vi "REST_req.vi"(5 "Request":T2(ring), 6 "Multipart Data In":T1[](array[typedef])=[{"Name"="imageblock1", "Value"="Collectable", "File"=path "C:/Users/monke/Desktop/Work/VIs to modify/ONENOTE/Sandbox/curl-logo.png", "Filename"="curl-logo.png", "MIME type"="image/png"}, {"Name"="content", "Value"="swagmaster flash", "File"=path "", "Filename"="Nothing", "MIME type"="image/png"}], 7 "Headers":string, 8 "error in":errorcluster, 9 "Body":string, 10 "Content-Type":string, 11 "URL":string) -> (0 "error out":errorcluster, 2 "ERROR":string, 3 "OUTPUT":string)   [LabVIEW 2016]
uses:
  <vilib>/httpClient/MultipartData.ctl
  <vilib>/httpClient/LabVIEWHTTPClient.lvlib
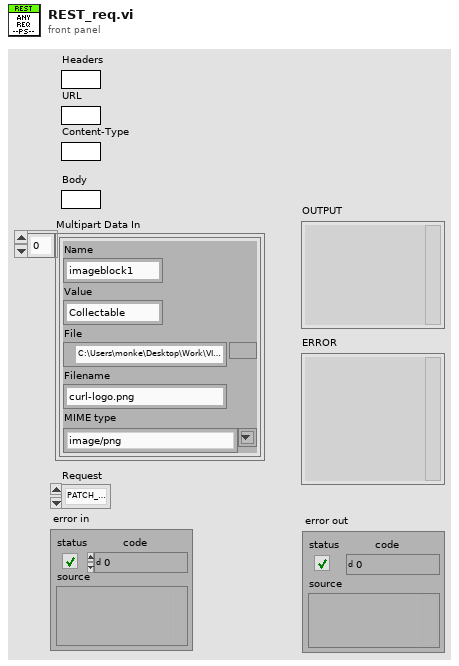
[diagram p1: front panel]
types:
  T1 = typedef "LabVIEWHTTPClient.lvlib/MultipartData.ctl" = cluster{"Name":string, "Value":string, "File":path, "Filename":string, "MIME type":string}
  T2 = enum16{"PATCH_MULTIPART", "POST_MULTIPART", "PATCH", "DELETE", "HEAD", "PUT", "GET"}
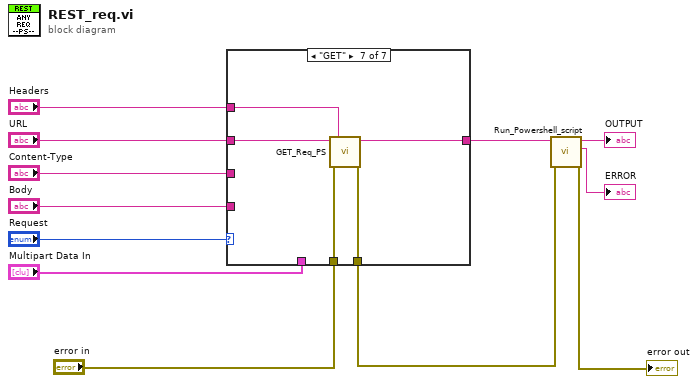
[diagram p0: block diagram]
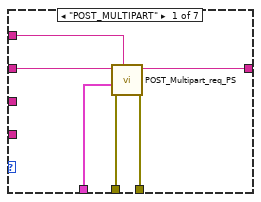
[diagram p2: hidden frame]
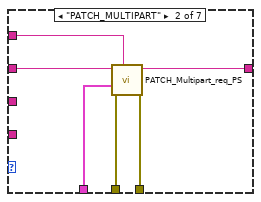
[diagram p3: hidden frame]
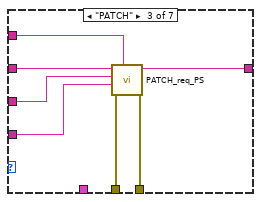
[diagram p4: hidden frame]
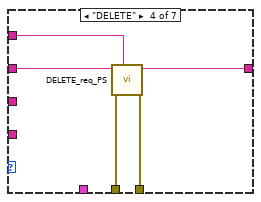
[diagram p5: hidden frame]
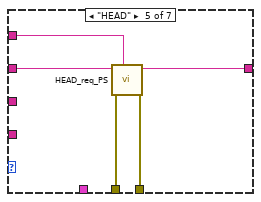
[diagram p6: hidden frame]
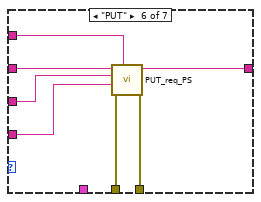
[diagram p7: hidden frame]
diagram:
  n1 = case shown="\"GET\"" "Request" {
    tunnel: "Multipart Data In" -> [w18 w24 _ _ _ _ _]
    tunnel: "URL" -> [w15 w23 w31 w33 w39 w48 w50]
    tunnel: "error in" -> [w17 w19 w30 w36 w41 w45 w51]
    tunnel: [w16 w20 w29 w35 w40 w44 w52] -> w5
    tunnel: "Headers" -> [w14 w22 w28 w32 w38 w43 w49]
    tunnel: [w13 w21 w25 w34 w37 w42 w53] -> w6
    tunnel: "Content-Type" -> [_ _ w26 _ _ w47 _]
    tunnel: "Body" -> [_ _ w27 _ _ w46 _]
    frame "POST_MULTIPART" {
      n2 = call "POST_Multipart_req_PS.vi"("Headers"=w14, "error in"=w17, "Multipart Data In"=w18, "URL"=w15) -> ("error out"=w16:errorcluster, "Multipart PATCH Request"=w13:string)  [unwired: 6 in]
    }
    frame "PATCH_MULTIPART" {
      n3 = call "PATCH_Multipart_req_PS.vi"("Headers"=w22, "error in"=w19, "Multipart Data In"=w24, "URL"=w23) -> ("error out"=w20:errorcluster, "Multipart PATCH Request"=w21:string)  [unwired: 6 in]
    }
    frame "PATCH" {
      n4 = call "PATCH_req_PS.vi"("Headers"=w28, "error in"=w30, "Body"=w27, "ContentType"=w26, "URL"=w31) -> ("error out"=w29:errorcluster, "PATCH Request"=w25:string)  [unwired: 5 in]
    }
    frame "DELETE" {
      n5 = call "DELETE_req_PS.vi"("Headers"=w32, "error in"=w36, "URL"=w33) -> ("error out"=w35:errorcluster, "DELETE Request"=w34:string)  [unwired: 7 in]
    }
    frame "HEAD" {
      n6 = call "HEAD_req_PS.vi"("Headers"=w38, "error in"=w41, "URL"=w39) -> ("error out"=w40:errorcluster, "HEAD Request"=w37:string)  [unwired: 7 in]
    }
    frame "PUT" {
      n7 = call "PUT_req_PS.vi"("Headers"=w43, "error in"=w45, "ContentType"=w46, "Body"=w47, "URL"=w48) -> ("error out"=w44:errorcluster, "PUT Request"=w42:string)  [unwired: 5 in]
    }
    frame "GET" {
      n8 = call "GET_Req_PS.vi"("Headers"=w49, "error in"=w51, "URL"=w50) -> ("error out"=w52:errorcluster, "GET Request"=w53:string)  [unwired: 7 in]
    }
  }
  n9 = call "Run_Powershell_script.vi"("error in"=w5, "Powershell Script"=w6) -> ("error out"=→"error out":errorcluster, "standard error"=→"ERROR":string, "standard output"=→"OUTPUT":string)  [unwired: 7 in]
